vi "AlliGator All ROIs Phasor Analysis.vi"(8 "error in (no error)":errorcluster, 10 "New Plot Name":string, 11 "AlliGator Internal Variables DVR":refnum<data-value>) -> (0 "error out":errorcluster, 1 "Calibrated Phasor":T1, 2 "Phasor Plot":cluster{"g Array":dbl[], "s Array":dbl[]}, 3 "AlliGator Internal Variables DVR":refnum<data-value>, 4 "Calibrated Phase Lifetime":dbl[unit], 6 "Message":string)   [LabVIEW 2021, in "AlliGator Phasor Graph.lvlib"]
doc: "Non-interactive phasor analysis of all ROIs."
uses:
  AlliGator Phasor Graph.lvlib
  Internal Variables/AlliGator Internal Variables v2.ctl
  <vilib>/vision/Image Controls.llb/IMAQ Image.ctl
  Internal Variables/AlliGator Gate Image Set.ctl
  Files/AlliGator FLI Dataset Type.ctl
  Files/AlliGator Data Series Type.ctl
  Dual-Channel Datasets/AlliGator Dataset Channel.ctl
  Settings/AlliGator Gate Arithmetic.ctl
  Source Image/AlliGator Displayed Image.ctl
  Image/Named ROI Description.ctl
  AlliGator Decay Metadata v3.ctl
  Decay Analysis/Decay Preprocessing/AlliGator Decay Background Subtraction Info.ctl
  Decay Analysis/Decay Preprocessing/AlliGator Baseline Subtraction Method.ctl
  Graphs/XY Graph/XY Graph Plot Shift Parameters.ctl
  Graphs/XY Graph/XY Graph Plot Shift Method.ctl
  Decay Analysis/Decay Preprocessing/AlliGator Decay Extrapolation Parameters.ctl
  Phasor/Calibration Phasor (m, phi).ctl
  Phasor/Phasor Reference Series.ctl
  Phasor/Phasor Calibration Map v2.ctl
  Phasor/Phasor (g, s).ctl
  AlliGator Raw Phasor Plot Data v5.ctl
  Phasor/Phasor Standard Deviation Options.ctl
  Phasor Plot/AlliGator Phasor Multi-Harmonic Data.ctl
  Phasor/Phasor Harmonic Data.ctl
  Decay Fit Parameter Map/AlliGator Decay Fit Options & Parameters v4.ctl
  Fits/IRF(X)PSED/Decay Fit Options v4.ctl
  Fits/Decay Convolution/Decay Model.ctl
  Fits/Residual Type.ctl
  Fits/IRF(X)PSED/Fit Weights Type v2.ctl
  Fits/Non-linear Fitting Method v2.ctl
  Fits/Fit Calculation Method.ctl
  Fits/Non-linear Fitting Algorithm.ctl
  Decay Analysis/Decay Fit/AlliGator Decay Fit Parameter Constraints 2.ctl
  Fits/IRF(X)PSED/Decay Fit Parameters In List.ctl
  Fits/IRF(X)PSED/MLE Baseline Offset Type.ctl
  Decay Analysis/Decay Preprocessing/AlliGator Decay Preprocessing Parameters.ctl
  Fits/IRF(X)PSED/Decay Fit Parameters & Derived Quantities List v2.ctl
  Fits/IRF(X)PSED/Decay Fit Result Constraint.ctl
  Decay Fit Parameter Map/AlliGator Parameter Maps Data.ctl
  Globals, Variables, Constants/AlliGator Variables List.ctl
  Settings/AlliGator Settings List.ctl
  Rich Text Box/Text Format List.ctl
  Variant/Variant to Data/Variant to U16.vi
  <vilib>/Utility/error.llb/Error Cluster From Error Code.vi
  Globals, Variables, Constants/AlliGator Abort.vi
  <vilib>/ErrorRing/Error Ring.xnode
  Globals, Variables, Constants/AlliGator Globals, Variables & Constants.lvlib
  Image/Image.lvlib
  Decay Analysis/Decay Processing/AlliGator Decay Processing.lvlib
  Source Image/AlliGator Source Image.lvlib
  Phasor Calibration/AlliGator Phasor Calibration.lvlib
  Settings/AlliGator Settings.lvlib
  Phasor/Phasor.lvlib
  Strings/Strings.lvlib
  Time/Time.lvlib
  Decay Analysis/Decay Preprocessing/AlliGator Decay Preprocessing.lvlib
  Graphs/XY Graph/XY Graph Add-Ons.lvlib
  GUI/GUI.lvlib
  Notebook/Notebook.lvlib
  Error/Error.lvlib
  Variant/Variant to Data/Variant to Data.lvlib
  Utilities/Utilities.lvlib
  Files/AlliGator Files.lvlib
  Internal Variables/AlliGator Internal Variables.lvlib
  Phasor Plot/AlliGator Phasor Plot.lvlib
  Fits/Fits.lvlib
  Decay Analysis/Decay Fit/AlliGator Decay Fit.lvlib
  Dual-Channel Datasets/AlliGator Dual-Channel Datasets.lvlib
  Decay Fit Parameter Map/AlliGator Decay Fit Parameter Map.lvlib
panel:
  # "see the AlliGator License on the block diagram (Ctrl+E or Window:Show Block Diagram)"
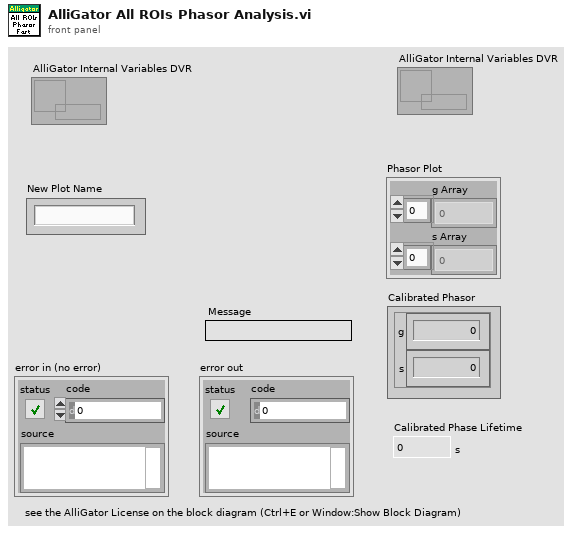
[diagram p1: front panel]
types:
  T1 = typedef "Phasor.lvlib/Phasor (g, s).ctl" = cluster{"g":dbl, "s":dbl}
  T2 = typedef "Phasor.lvlib/Phasor Standard Deviation Options.ctl" = cluster{"Compute Estimated SDV":bool, "# Replicas":u32, "Use Estimated Average Phasor":bool}
  T3 = typedef "AlliGator Settings.lvlib/AlliGator Settings List.ctl" = enum16{"GUI:Visible Settings Tab", "GUI:Last Run Version", "Source Image:Use Image Histogram for Contrast", "Source Image:Low Count Pixels Rejection Options", "Source Image:High Count Pixels Rejection Options", "Source Image:Use Image Brightness", "Source Image:Blend Overlay with Image Background", "Source Image:Use Fixed ROI Diameter", "Source Image:ROI Diameter", "Source Image:ROI Center Color", "Source Image:Peak Threshold", "Source Image:Intensity Threshold", "Source Image:Image Binning Options", "Source Image:Image Smoothing Options", "Source Image:Image Histogram Active", "Source Image:Invert Binary Mask", "Source Image:Hot Pixel Removal", "Source Image:Overlay Analyzed ROI Center", "Source Image:Auto-Adjust Contrast", "Source Image:Histogram Lower Percentile", "Source Image:Histogram Upper Percentile", "Source Image:Save Source Image", "Source Image:Scale Bar Options", "Source Image:Image Resolution (Pixel Size)", "Source Image:Flatfield Correction", "Source Image:Show Dead Left Columns Correction", "Source Image:Dead Left Columns Correction", "Source Image:Image Pre-Processing Operations Order", "Source Image:Overlay ROI Median", "Source Image:Median Overlay Color", "Data Information:Gate Width", "Data Information:Nanotime Gate Separation", "Data Information:Macrotime Gate Separation", "Data Information:Gate Step", "Data Information:# Gates", "Data Information:Gate Image Exposure", "Data Information:Gate Image Integration", "Data Information:Gates to Skip", "Data Information:Gates to Keep", "Data Information:Define Gates to", "Data Information:Channel Name", "Data Information:Available Channel Names", "Data Information:Channel Arithmetic", "Data Information:Background File Subtraction", "Data Information:Background File", "Data Information:Background Scaling Factor", "Data Information:Background Pile-up Correction", "Data Information:Background Pixel Well Capacity", "Data Information:Laser Period", "Data Information:SYNC Period", "Data Information:Pile-up Correction", "Data Information:Pixel Well Capacity", "Data Information:Dataset Scaling Factor", "Fluorescence Decay_Decay Pre-Processing:Reverse Gates", "Fluorescence Decay_Decay Pre-Processing:Verbose Decay Pre-Processing", "Fluorescence Decay_Decay Pre-Processing:Use Decay Pre-Processing", "Fluorescence Decay_Decay Pre-Processing:Background Subtraction", "Fluorescence Decay_Decay Pre-Processing:Background Definition Range", "Fluorescence Decay_Decay Pre-Processing:Baseline Subtraction Method", "Fluorescence Decay_Decay Pre-Processing:Decay Pre-Processing Operations Order", "Fluorescence Decay_Decay Pre-Processing:Smoothing Parameter", "Fluorescence Decay_Decay Pre-Processing:Shift Decay", "Fluorescence Decay_Decay Pre-Processing:Decay Shift Parameters", "Fluorescence Decay_Decay Pre-Processing:Fold Decay", "Fluorescence Decay_Decay Pre-Processing:# Folds", "Fluorescence Decay_Decay Pre-Processing:1-Normalize Decay", "Fluorescence Decay_Decay Pre-Processing:[0-1]-Normalize Decay", "Fluorescence Decay_Decay Pre-Processing:Smoothen Decay", "Fluorescence Decay_Decay Pre-Processing:Extrapolate Decay", "Fluorescence Decay_Decay Pre-Processing:Use Periodicity", "Fluorescence Decay_Decay Pre-Processing:Use Cursors", "Fluorescence Decay_Decay Pre-Processing:Tail Fraction", "Fluorescence Decay_Decay Pre-Processing:Head Fraction", "Fluorescence Decay_Decay Pre-Processing:Additional Points", "Fluorescence Decay_Decay Pre-Processing:Straighten Decay", "Fluorescence Decay_Decay Pre-Processing:Constant Background", "Fluorescence Decay_Decay Pre-Processing:Pixel-Normalize Decay", "Fluorescence Decay_Advanced Analysis:Extract IRF instead of Decay", "Fluorescence Decay_Advanced Analysis:IRF Extraction Options", "Fluorescence Decay_Advanced Analysis:IRF Optimization Options", "Fluorescence Decay_Advanced Analysis:Square Pulse Options", "Fluorescence Decay_Advanced Analysis:IRF Order", "Fluorescence Decay_Advanced Analysis:IRF Time Constants", "Fluorescence Decay_Advanced Analysis:Wavelet Analysis Options", "Fluorescence Decay_Advanced Analysis:Average Lifetime Options", "Fluorescence Decay_Fit Options:Fit Options", "Fluorescence Decay_Fit Options:Use Legacy Fitting Approach", "Fluorescence Decay_Fit Options:Use Data Information Laser Period", "Fluorescence Decay_Fit Parameters:Displayed Fit Parameters", "Fluorescence Decay_Fit Parameters:Fit Parameter Constraints", "Fluorescence Decay_Fit Parameters:Export Tabulated Results", "Fluorescence Decay_Fit Parameters:MLE Baseline Offset Type", "Fluorescence Decay_Fit Parameters:MLE Baseline Offset", "Fluorescence Decay_Fit Parameters:Guess Parameter Names", "Fluorescence Decay_Fit Parameters:Guess Parameter Values", "Fluorescence Decay_Fit Parameters:Guess Parameters Options", "Fluorescence Decay_Fit Parameters:Optimal Offset Selection Criterion", "Fluorescence Decay_Styles:Show Last Decay Only", "Fluorescence Decay_Styles:Decay Graph Color Array", "Fluorescence Decay:Decay Graph Active", "Fluorescence Decay Statistics:Min Peak Value", "Fluorescence Decay Statistics:Reject Low Decay Peak Pixels", "Fluorescence Decay Statistics:Reject High Decay Peak Pixels", "Fluorescence Decay Statistics:Max Peak Value", "Time Traces:Use File Timestamp", "Time Traces:Time Step", "Time Traces:Use Intensity Correction File", "Time Traces:Intensity Correction File", "Phasor Plot:Phasor Plot Smoothing Options", "Phasor Plot:Phasor Plot Size", "Phasor Plot:Phasor Plot Graphics Options", "Phasor Plot:Cumulative Phasor Plot", "Phasor Plot:Use Phasor Brightness", "Phasor Plot:Blend Overlay with Phasor Background", "Phasor Plot:Save Phasor Plot", "Phasor Plot:Show References", "Phasor Plot:Phasor Ratio Decay Range", "Phasor Plot:Exponential Fading", "Phasor Plot:Phasor Ratio Reference Colors", "Phasor Plot:Reference Radius", "Phasor Plot:Show Color Map Vertices", "Phasor Plot:Phasor Plot Active", "Phasor Plot:Phasor Ratio Color Map Type", "Phasor Plot:Phasor Ratio Color Map", "Phasor Plot:Phasor Ratio Display Range", "Phasor Plot:Selected Image ROI(s)", "Phasor Plot:All Image ROIs", "Phasor Plot:Selected Phasor Plot ROI(s)", "Phasor Plot:All Phasor Plot ROIs", "Phasor Plot:Phasor Ratio Color-Coded Quantity", "Phasor Plot:Store Phasor Harmonics", "Phasor Plot:Draw Reference Segment", "Phasor Plot:User-Defined Quantity", "Phasor Plot:Color Scale High Color", "Phasor Plot:Color Scale Low Color", "Phasor Plot:Intensity-weighted Phasor Plot", "Phasor Graph:Phasor Frequency", "Phasor Graph:Phasor Ratio Type", "Phasor Graph:Pixel-level Phasor Computation", "Phasor Graph:Save Phasor Graph", "Phasor Graph:Phasor Graph Active", "Phasor Graph:Phasor SDV Options", "Phasor Graph:Intensity-weighted Phasor Graph", "Phasor Graph:Define Shortest Lifetime as", "Phasor Calibration:Use Backup Calibration if needed", "Phasor Calibration:Backup Calibration Type", "Phasor Calibration:Calibration Type", "Phasor Calibration:Calibration Lifetime", "Phasor Calibration:Calibration Map Algorithm", "Single-Exponential Phasor Locus (SEPL):Gate Parameters", "Single-Exponential Phasor Locus (SEPL):User-defined Gate", "Single-Exponential Phasor Locus (SEPL):User-defined IRF", "Single-Exponential Phasor Locus (SEPL):Phasor Parameters", "Single-Exponential Phasor Locus (SEPL):Decay & IRF Parameters", "Single-Exponential Phasor Locus (SEPL):Display Parameters", "Lifetime Analysis:Decay Analysis Parameters", "Lifetime Analysis:Lifetime Map Active", "Plugins:Python Settings", "Miscellaneous:Verbose Mode", "Miscellaneous:Beep after Script", "Miscellaneous:Saved Image File Format", "Miscellaneous:Exported Gate Image Settings", "Miscellaneous:Include Loading in Timing", "Miscellaneous:Verbose Settings Mode", "Miscellaneous:Histogram Options", "Miscellaneous:Beep on Error", "Miscellaneous:# Logical Processors Used", "Miscellaneous:ROI Description Max Characters", "Miscellaneous:Verbose Error Mode", "Miscellaneous:Transparent Mask Color"}
  T4 = typedef "AlliGator Globals, Variables & Constants.lvlib/AlliGator Variables List.ctl" = enum16{"---- GUI ----", "GUI:Initialization Status", "GUI:State Indicators Refnum", "GUI:Original AlliGator Menu Items", "GUI:Current Action Loop State", "GUI:Script in progress", "GUI:Playback", "GUI:Loop Playback", "GUI:Search ROI Used", "GUI:Search ROI", "Decay Graph Max Legend Size", "Intensity Graph Max Legend Size", "Decay Statistics Graph Max Legend Size", "Phasor Graph Max Legend Size", "Phasor Ratio Graph Max Legend Size", "Lifetime Graph Max Legend Size", "---- Files ----", "Files:Export Dataset Frames as Individual Files", "Files:Show Batch Export Help Balloons", "Files:Frames in Dataset", "Files:ptu File Frame Start Indices", "Files:Current Frame in Dataset", "Files:Current Frame Timestamp", "Files:Dataset Loaded", "Files:Dataset Metadata", "Files:Dataset Channel", "Files:Dataset Data Description", "Files:Background Dataset Metadata", "Files:Background Dataset Channel", "Files:Background Dataset Data Description", "Files:Background File Subtraction", "Files:Background File Path", "Files:Background File Pile-up Correction", "Files:Background File Pixel Well Capacity", "Files:Background File Scaling Factor", "Files:Current Dataset Load Settings", "Files:Dataset Path", "Files:ICCD-specific Information", "Files:Macrotime Gate Separation", "------ Python Plugins ------", "Python Plugins:Information", "Python Plugins:Python Session", "Python Plugins:Valid Python Session?", "---- Source Image ----", "Source Image:ROIs", "Source Image:Current ROI", "Source Image:ROI Event Refnum", "X_Source Image:Display Range", "X_Source Image:Palette Information", "X_Source Image:Type of Displayed Image", "X_Time Gate Slider", "Source Image:Palette List", "Source Image:Scale", "Source Image:ROI Overlay Color", "Source Image:Overlay to Erase", "Source Image:Is Displayed Image Accumulated", "Source Image:White Light Image Modified", "Source Image:Mask Image Modified", "---- Image Profile Window ----", "Image Profile:Window Event Refnum", "Image Profile:IntensityType", "Image Profile:Intensity Average Type", "Image Profile:Intensity-weighted SDV", "Image Profile:Box Profile Type", "Image Profile:Window Open", "Image Profile:Plotted Fit Parameter", "------ Phasor Graph -------", "Phasor Graph:Show Line", "---- Phasor Plot ---", "Phasor Plot:Parameters Changed", "Phasor Plot:FLI Dataset Modified since last Calculation", "Phasor Harmonics Data", "Selected Phasor Harmonics", "Phasor Harmonic Manager Event Refnum", "Phasor Plot:ROIs", "Phasor Plot:Current ROI", "Phasor Plot:ROI Event Refnum", "Phasor Plot:Image Reference Points", "Phasor Plot:Computed", "Phasor Plot:Palette Information", "Phasor Plot:Palette List", "Phasor Plot:Phasor Ratio Palette Information", "Phasor Plot:Phasor Ratio Palette List", "Phasor Plot:Image Scale", "Phasor Plot:Image Overlay to Erase", "Phasor Plot:Image Elements to Update", "Phasor Plot:Current Calculation Parameters", "Phasor Plot:Current Calibration Options", "Phasor Plot:Reset Cumulated Phasor Plot", "Phasor Plot:Reference 1", "Phasor Plot:Lifetime Reference 1", "Phasor Plot:Reference 1 Frequency", "Phasor Plot:Reference 2", "Phasor Plot:Lifetime Reference 2", "Phasor Plot:Reference 2 Frequency", "---- Decay Analysis ----", "Number of Selected Decays to Fit", "LS Fit Results", "LAR Fit Results", "BS Fit Results", "Last Decay Max - Min", "Best Fit Parameters", "Best Fit Parameter Names", "Actual Size X", "Actual Size Y", "Binning X", "Binning Y", "Actual # Gates", "Dataset Number", "Gates to...", "Gates Skipped", "Gates to keep", "Gate Step", "Gate Separation", "Reversed Gates", "Pile-up Correction", "Pixel Well Capacity", "Background Subtracted", "Background Subtraction Method", "Background Definition Range", "Background File (deprecated)", "Number of Dataset Accumulated", "Array of Accumulated Dataset Paths", "Do Averaged Datasets", "Destination File Path", "Process Plot Target", "Use 1/D as Phasor Frequency", "---- Decay Fit Parameter Map -----", "Decay Fit Parameter Map:Palette Information", "Decay Fit Parameter Map:Palette List", "Decay Fit Parameter Map:X Resolution", "Decay Fit Parameter Map:Y Resolution", "Decay Fit Parameter Map:Use Decay Fit Result Constraints", "Decay Fit Parameter Map:Decay Fit Result Constraints", "Decay Fit Parameter Map:Decay Fit Result Constraints Applied", "---- Parameter Map ----", "Parameter Map:Palette Information", "Parameter Map:Palette List", "------- Local Decay Window ---------", "Local Decay Graph Window:Event Refnum", "Local Decay Graph Window:Use normalized IRF for convolution", "----- Miscellaneous ----", "Misc:Skippable Dialog Windows Status"}
  T5 = typedef "IMAQ Image.ctl" = refnum<image>
  T6 = typedef "Image.lvlib/Named ROI Description.ctl" = cluster{"ROI Descriptor":T7, "ROI Name":string, "Overlay Color":u32}
  T7 = typedef "ROI Descriptor" = cluster{"Global Rectangle":i32[], "Contours":cluster{"ID":enum32{"External", "Internal"}, "Type":u32, "Coordinates":i32[]}[]}
  T8 = typedef "Notebook.lvlib/Text Format List.ctl" = enum16{"Message", "Result", "Error", "Setting", "Verbose", "Warning"}
  T9 = typedef "AlliGator Phasor Graph.lvlib/AlliGator Raw Phasor Plot Data v5.ctl" = cluster{"Phasor Plot Name":string, "Raw Phasor Plot":T1[], "Phasor Frequency":dbl[unit], "[Decay Metadata]":T10[], "Raw Phasor Plot SDV":T1[], "Phasor SDV Options":T2, "[Calibration Phasor]":T16[], "Intensity Array":dbl[]}
  T10 = typedef "AlliGator Phasor Graph.lvlib/AlliGator Decay Metadata v3.ctl" = cluster{"ROI Descriptor":T7, "ROI Center":cluster{"X":i32, "Y":i32}, "Decay Background Subtraction Info":T11, "Decay Reverted":bool, "Decay Smoothened":bool, "Decay Straightened":bool, "Fitted Tau (Decay Straightening)":dbl, "Decay Shift Parameters":T13, "Decay Shifted":bool, "Decay Extrapolated":bool, "Decay Extrapolation Parameters":T15, "Decay Normalized":bool, "Fold Decay":bool, "# Folds":u32}
  T11 = typedef "AlliGator Decay Preprocessing.lvlib/AlliGator Decay Background Subtraction Info.ctl" = cluster{"Laser Period":dbl[unit], "Gate Duration":dbl[unit], "Baseline Subtraction Method":T12, "Background Definition Range":cluster{"Min Gate":dbl[unit], "Max Gate":dbl[unit]}, "Total Intensity w/o Bkgd Subtraction":dbl, "Bkgd-subtracted Intensity (exp)":dbl, "# Data Points":i32, "Background/Gate":dbl, "Fitted Lifetime":dbl[unit], "Bkgd-subtracted Intensity (theo)":dbl}
  T12 = typedef "AlliGator Decay Preprocessing.lvlib/AlliGator Baseline Subtraction Method.ctl" = enum16{"Mean", "Min", "Square Gated Single-Exponential", "File", "Constant"}
  T13 = typedef "XY Graph Add-Ons.lvlib/XY Graph Plot Shift Parameters.ctl" = cluster{"Type":T14, "Shift":dbl[unit], "Threshold":dbl, "Rotate":bool}
  T14 = typedef "XY Graph Add-Ons.lvlib/XY Graph Plot Shift Method.ctl" = enum16{"Default", "CFD", "Threshold", "Cross-Correlation"}
  T15 = typedef "AlliGator Decay Preprocessing.lvlib/AlliGator Decay Extrapolation Parameters.ctl" = cluster{"Additional Points":u32, "Head Fraction":dbl, "Fitted Tau":dbl, "Use Periodicity":bool, "Use Cursors":bool, "Tail Fraction":dbl}
  T16 = typedef "Phasor.lvlib/Calibration Phasor (m, phi).ctl" = cluster{"m":dbl, "phi":dbl, "Phasor Frequency":dbl[unit], "Reference Lifetime":dbl[unit]}
  T17 = typedef "AlliGator Internal Variables.lvlib/AlliGator Internal Variables v2.ctl" = cluster{"----------------------------- Images -----------------------------":u8, "Displayed Image":T5, "White Light Image":T5, "Mask Image":T5, "ROI Mask Image":T5, "Current Dataset Images 1":T18, "Background Dataset Images 1":T18, "Current Dataset Images 2":T18, "Background Dataset Images 2":T18, "Current Dataset Arithmetic Images":T18, "Accumulated Dataset Images 1":T18, "Accumulated Dataset Images 2":T18, "Accumulated Dataset Arithmetic Images":T18, "----------------------------- File Paths -----------------------------":u8, "Phasor Plot Image":T5, "Decay Fit Parameter Map Image":T5, "Parameter Map Image":T5, "Single Data Point Path":path, "White Light Image Path":path, "Mask Image Path":path, "Time-Series Folder":path, "[Time-Series Paths]":path[], "----------------------------- FLI Dataset -----------------------------":u8, "Current Dataset":i32, "Single Dataset Type":T19, "Current Folder":string, "AlliGator Data Series Type":T20, "# Datasets":i32, "Dual-Channel Dataset":bool, "Selected Channel Name":string, "Dataset Channel":T21, "Channel Arithmetic":T22, "Dual-Channel Background Dataset":bool, "Background Channel":T21, "Dual-Channel Accumulated Dataset":bool, "Start Time":dbl, "[Time-Series Timestamps]":dbl[], "[Intensity Corrections]":dbl[], "Time Series Script":bool, "Type of Displayed Image":T23, "Gate Image Slide":u16, "# Gates":i32, "ROIs":T6[], "----------------------------- Decays -----------------------------":u8, "ROI Decay":cluster{"t Array":dbl[], "I Array":dbl[]}, "Valid Decay":bool, "Decay  Metadata":T10, "Reference Decay Plot Name":string, "Reference Decay":cluster{"t Array":dbl[], "I Array":dbl[]}, "Decay Shift Plot":cluster{"Time Stamps":dbl[], "Decay Shifts":dbl[]}, "[Decays Max Values]":sgl[], "[Decays Min Values]":sgl[], "----------------------------- Calibration -----------------------------":u8, "Calibration Phasor":T16, "Calibration Phasor Series":T24, "Phasor Calibration Map":T25, "Calibration Map MD5 Digest":string, "----------------------------- Phasor Graph -----------------------------":u8, "Last Raw Phasor":T1, "Last Calibrated Phasor":T1, "Last Calibrated Phasor SDV":T1, "Phasor Graph:Phasor Plot":cluster{"g Array":dbl[], "s Array":dbl[]}, "Phasor Graph:Phasor SDV Plot":cluster{"g Array":dbl[], "s Array":dbl[]}, "[Phasor Graph:Raw Phasor Plots]":T9[], "Phasor Plot locked to Ref 1":i32, "[Phasor Plot(s) locked to Ref 1]":i32[], "[Phasor Plot(s) locked to Ref 2]":i32[], "[Pixel Phasors]":T1[], "----------------------------- Phasor Plot -----------------------------":u8, "[[Sum Image]]":dbl[][], "[[CSG Phasors]]":csg[][], "[[Valid Pixel?]]":bool[][], "[[Phasor Ratios]]":dbl[][], "[[Average Lifetimes]]":dbl[][], "Amplitude Weighted Average Lifetime":bool, "I/m/phi Dataset":cluster{"I/m/phi Dataset?":bool, "Base Frequency":dbl[unit], "Harmonic Orders":u8[]}, "Multi Phasor Plot Data":T26, "----------------------------- Decay Fit Parameter Map -----------------------------":u8, "Decay Fit Options & Parameters":T28, "Fit Options: Decay Preprocessing Parameters":T39, "Fit Options: Reference Decay":cluster{"t Array":dbl[], "I Array":dbl[]}, "Is Full Image Parameters Map":bool, "Is Single-Pixels Parameters Map":bool, "NLSF Parameters Map X Resolution":i32, "NLSF Parameters Map Y Resolution":i32, "[Single Decay Fit Parameters]":dbl[], "Fit Model":T30, "[[Multiple Decays Fit Parameters]]":dbl[][], "[[Multiple Decays Fit Parameter SDVs]]":dbl[][], "[[IRFs]]":dbl[][], "[ROI Descriptors]":T7[], "IRF Array Time Axis":dbl[], "Decay Array Time Axis":dbl[], "[Decay Fit Parameter Names]":T40[], "[Decay Sum]":dbl[], "Array of Decay Fit Result Constraints":T41[], "Selected ROIs Array":bool[], "----------------------------- Parameter Maps -----------------------------":u8, "[Map Set Names]":string[], "[Parameter Maps]":T42[], "[[User-defined Quantities]]":dbl[][], "User-defined Quantity":string}
  T18 = typedef "AlliGator Internal Variables.lvlib/AlliGator Gate Image Set.ctl" = cluster{"SGL Gate Images":T5[], "SGL Sum Image":T5, "SGL Max Image":T5, "SGL Min Image":T5}
  T19 = typedef "AlliGator Files.lvlib/AlliGator FLI Dataset Type.ctl" = enum16{"HDF5 FLI Dataset", "Gate Image Folder", ".sdt FLI Dataset (Becker & Hickl)", ".ptu FLI Dataset (PicoQuant)", "SS1 FLI Dataset", "SS2 FLI Dataset", "I/m/phi Dataset", ".bin FLI Dataset (PicoQuant Binned)", ".bin FLI Dataset (Piccolo Binned)", ".mat FLI Dataset"}
  T20 = typedef "AlliGator Files.lvlib/AlliGator Data Series Type.ctl" = enum16{"Not a Supported Series", "Gate Images Folder Series", "SwissSPAD 2 Dataset Series", "B&H FLI Dataset Series", "PicoQuant PTU FLI Dataset Series", "PicoQuant BIN FLI Dataset Series", "Piccolo hist BIN FLI Dataset Series", "HDF5 FLI Dataset Series"}
  T21 = typedef "AlliGator Dual-Channel Datasets.lvlib/AlliGator Dataset Channel.ctl" = enum16{"G2", "INT"}
  T22 = typedef "AlliGator Settings.lvlib/AlliGator Gate Arithmetic.ctl" = enum16{"None", "INT-G2", "G2/INT*<INT>", "(1 - G2/INT)*<INT>"}
  T23 = typedef "AlliGator Source Image.lvlib/AlliGator Displayed Image.ctl" = enum16{"Single Gate", "Sum of All Gates", "Max of All Gates", "Min of All Gates", "-", "White Ligth Image", "Mask Image"}
  T24 = typedef "Phasor.lvlib/Phasor Reference Series.ctl" = cluster{"m Array":dbl[], "phi Array":dbl[], "Phasor Frequency":dbl[unit], "Calibration Lifetime":dbl[unit]}
  T25 = typedef "Phasor.lvlib/Phasor Calibration Map v2.ctl" = cluster{"Phasor Frequency":dbl[unit], "Calibration Lifetime":dbl[unit], "ROI Centers":cluster{"X":i32, "Y":i32}[], "ROI Descriptors":T7[], "Map Resolution X":i32, "Map Resolution Y":i32, "z Array":cdb[]}
  T26 = typedef "AlliGator Phasor Plot.lvlib/AlliGator Phasor Multi-Harmonic Data.ctl" = cluster{"Base Frequency":dbl[unit], "# Harmonics":u8, "Harmonic Orders":u8[], "Phasor Plot Settings Checksum":u64, "Phasor Harmonic Data Array":T27[]}
  T27 = typedef "Phasor.lvlib/Phasor Harmonic Data.ctl" = cluster{"Phasor Harmonic Name":string, "Phasor Plot Settings Checksum":u64, "Phasor Frequency":dbl[unit], "Base Frequency":dbl[unit], "Harmonic Order":u8, "Phasor Plot Parameters":string, "Phasor Array [[CSG]]":csg[][], "Dataset File Path":path}
  T28 = typedef "AlliGator Decay Fit Parameter Map.lvlib/AlliGator Decay Fit Options & Parameters v4.ctl" = cluster{"SYNC Period":dbl[unit], "Fit Options":T29, "Fit Parameter Constraints":T36[], "MLE Baseline Offset":dbl, "MLE Baseline Offset Type":T38}
  T29 = typedef "Fits.lvlib/Decay Fit Options v4.ctl" = cluster{"Show Fit Residuals":bool, "Fit Model":T30, "Residual Type":T31, "Max Decay Percentile":dbl, "Min Decay Percentile":dbl, "Show Full Decay":bool, "Weights":T32, "Fitting Method":T33, "Compute Parameter Uncertainties":bool, "Periodic Boundaries":bool, "Model Calculation":T34, "Period":dbl[unit], "Termination Criteria":cluster{"Max Iterations":i32, "Max Function Calls":i32, "Max Time":dbl[unit], "Function Tolerance":dbl, "Parameter Tolerance":dbl, "Gradient Tolerance":dbl, "Min Lambda":dbl, "Max Lambda":dbl, "Initial Tick Count":u32}, "Offset Resolution":dbl[unit], "Use Local IRF":bool, "Fitting Algorithm":T35, "Show Confidence Interval ":bool, "Confidence Level":dbl}
  T30 = typedef "Fits.lvlib/Decay Model.ctl" = enum16{"1-Exponential", "2-Exponentials"}
  T31 = typedef "Fits.lvlib/Residual Type.ctl" = enum16{"Standard", "Normalized", "Reduced"}
  T32 = typedef "Fits.lvlib/Fit Weights Type v2.ctl" = enum16{"Unweighted", "1/Variance (Neyman)", "1/Variance (Pearson)", "Best of All"}
  T33 = typedef "Fits.lvlib/Non-linear Fitting Method v2.ctl" = enum16{"Least Square", "Least Absolute Residual", "Bisquare", "MLE", "-", "Best of All"}
  T34 = typedef "Fits.lvlib/Fit Calculation Method.ctl" = enum16{"Simulation", "Convolution", "Integration"}
  T35 = typedef "Fits.lvlib/Non-linear Fitting Algorithm.ctl" = enum16{"Levenberg-Marquardt", "Trust-Region Dogleg"}
  T36 = typedef "AlliGator Decay Fit.lvlib/AlliGator Decay Fit Parameter Constraints 2.ctl" = cluster{"Fit Parameter":T37, "Min Value":dbl, "Max Value":dbl, "Global":bool, "Used":bool}
  T37 = typedef "Fits.lvlib/Decay Fit Parameters In List.ctl" = enum16{"Offset", "Baseline", "A_1", "tau_1", "A_2", "tau_2"}
  T38 = typedef "Fits.lvlib/MLE Baseline Offset Type.ctl" = enum32{"Absolute", "Percentage"}
  T39 = typedef "AlliGator Decay Preprocessing.lvlib/AlliGator Decay Preprocessing Parameters.ctl" = cluster{"Background Subtraction":bool, "Straighten Decay":bool, "Reverse Gates":bool, "1-Normalized Decay":bool, "Smoothen Decay":bool, "Smoothing Parameter":dbl, "Shift Decay":bool, "Decay Shift Parameters":T13, "Extrapolate Decay":bool, "Additional Points":u32, "Head Fraction":dbl, "Pixel-Normalize Decay":bool, "Use Periodicity":bool, "Use Cursors":bool, "Tail Fraction":dbl, "Use Decay Pre-Processing":bool, "Fold Decay":bool, "# Folds":u32, "[0-1]-Normalized Decay":bool}
  T40 = typedef "Fits.lvlib/Decay Fit Parameters & Derived Quantities List v2.ctl" = enum16{"Offset", "Baseline", "A_1", "tau_1", "A_2", "tau_2", "<tau>_a", "f1_a", "f2_a", "<tau>_i", "f1_i", "f2_i", "-", "R^2", "Chi^2"}
  T41 = typedef "Fits.lvlib/Decay Fit Result Constraint.ctl" = cluster{"Fit Parameter":enum16{"Offset", "Baseline", "A_1", "tau_1", "A_2", "tau_2", "<tau>_a", "f1_a", "f2_a", "<tau>_i", "f1_i", "f2_i", "-", "R^2", "Chi^2", "Max Relative Residual", "<Residual ACF>", "Residual ACF SDV", "tau_2/tau_1"}, "Min Value":dbl, "Max Value":dbl, "Use Constraint":bool}
  T42 = typedef "AlliGator Decay Fit Parameter Map.lvlib/AlliGator Parameter Maps Data.ctl" = cluster{"Map Set Name":string, "[Parameter Names]":string[], "[[Parameters]]":dbl[][], "[[Parameter SDVs]]":dbl[][], "Decay Array Time Axis":dbl[], "[[IRFs]]":dbl[][], "IRF Array Time Axis":dbl[], "X Resolution":i32, "Y Resolution":i32, "Intensity Array":dbl[]}
  T43 = cluster{"Decay Peak Constraint":bool, "Min":dbl, "Max":dbl}
  T44 = typedef "Phasor.lvlib/Phasor Calibration Type.ctl" = enum16{"None", "Single Phasor", "Phasor Series", "Phasor Map"}
  T45 = cluster{"Use Backup Calibration if needed?":bool, "Calibration Type":T44}
  T46 = typedef "AlliGator Settings.lvlib/AlliGator Pixel Counts Constraints.ctl" = cluster{"High Count Pixels Rejection Options":T47, "Low Count Pixels Rejection Options":T48}
  T47 = typedef "AlliGator Settings.lvlib/AlliGator High Count Pixels Rejection Options.ctl" = cluster{"Background High Threshold Factor":dbl, "Fixed High Background Threshold":dbl, "Reject High Count Pixels":bool, "High Percentile":dbl}
  T48 = typedef "AlliGator Settings.lvlib/AlliGator Low Count Pixels Rejection Options.ctl" = cluster{"Background Low Threshold Factor":dbl, "Fixed Low Background Threshold":dbl, "Reject Low Count Pixels":bool, "Low Percentile":dbl}
  T49 = cluster{"t Axis":dbl[], "ROI Intensity Array":dbl[]}
  T50 = typedef "Rich Text Box.lvlib/Text Formatting.ctl" = cluster{"Font":string, "Text Color":T51, "Background Color":T51, "Style":T52, "Font Size":dbl, "Alignment":T53}
  T51 = typedef "Rich Text Box.lvlib/Text Colors.ctl" = enum16{"Unchanged", "Black", "Blue", "Cyan", "Maroon", "Gray", "Violet", "Green", "Light Green", "Orange", "Yellow", "Magenta", "Red", "White"}
  T52 = typedef "Rich Text Box.lvlib/Text Style.ctl" = enum16{"Regular", "Bold", "Italic", "Underline", "Strikeout"}
  T53 = typedef "Rich Text Box.lvlib/Text Alignment.ctl" = enum16{"Left", "Right", "Center"}
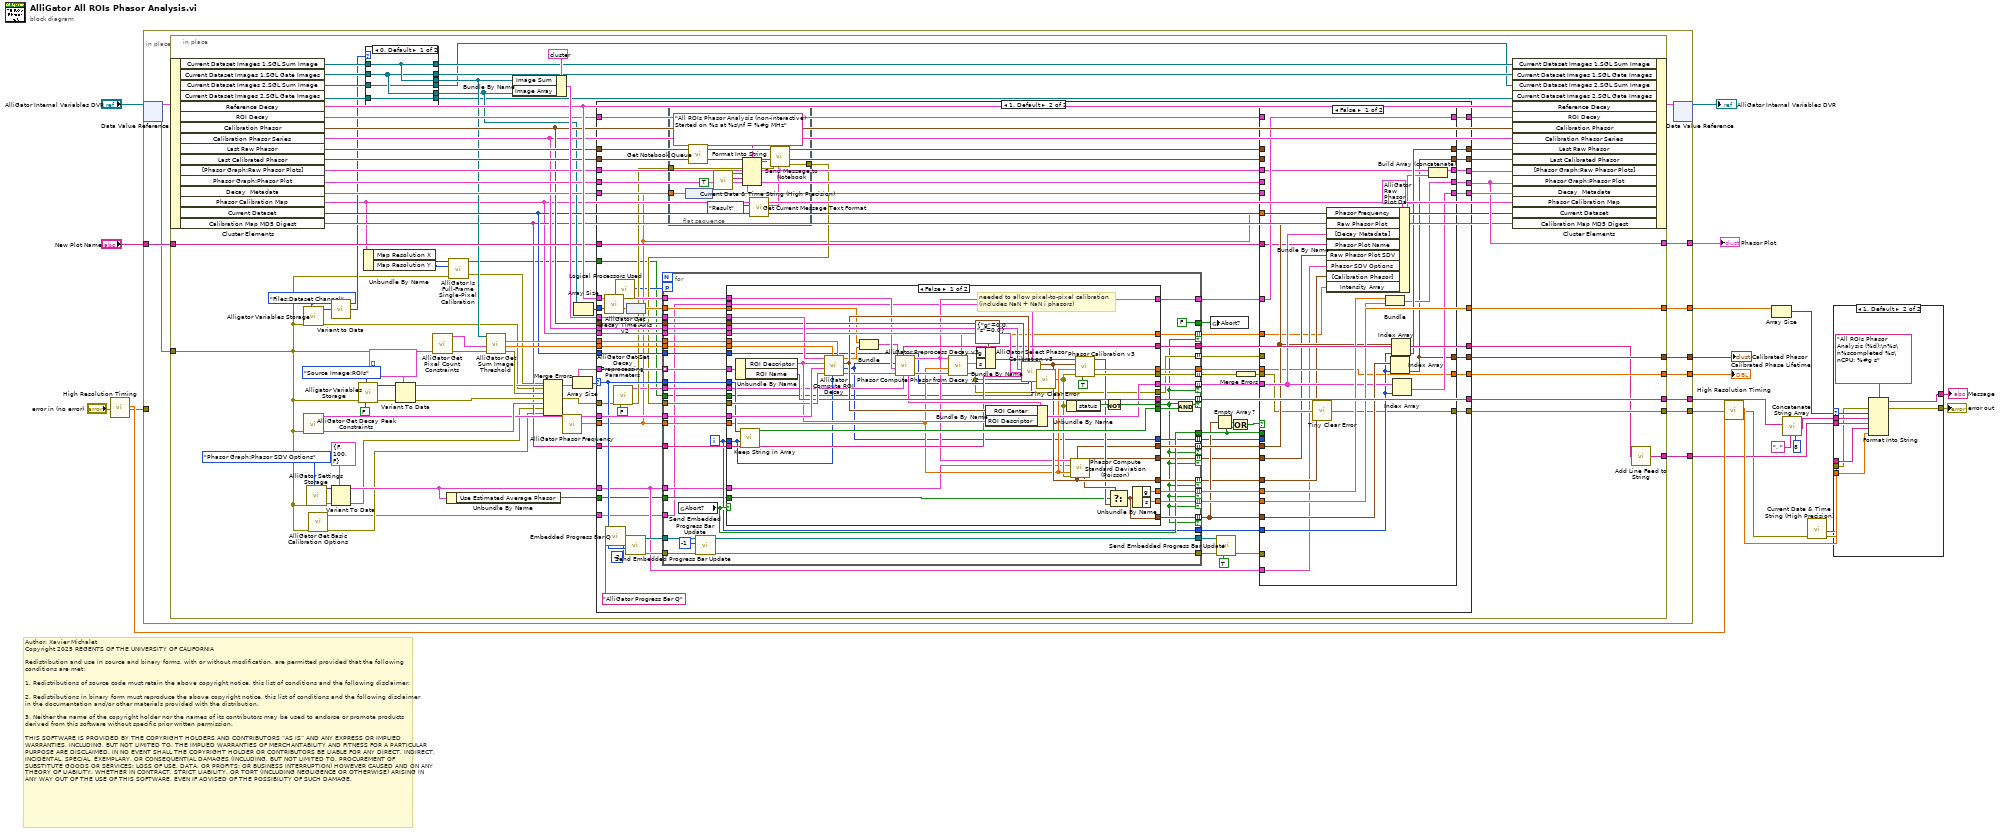
[diagram p0: block diagram]
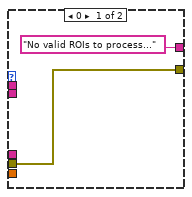
[diagram p2: hidden frame]
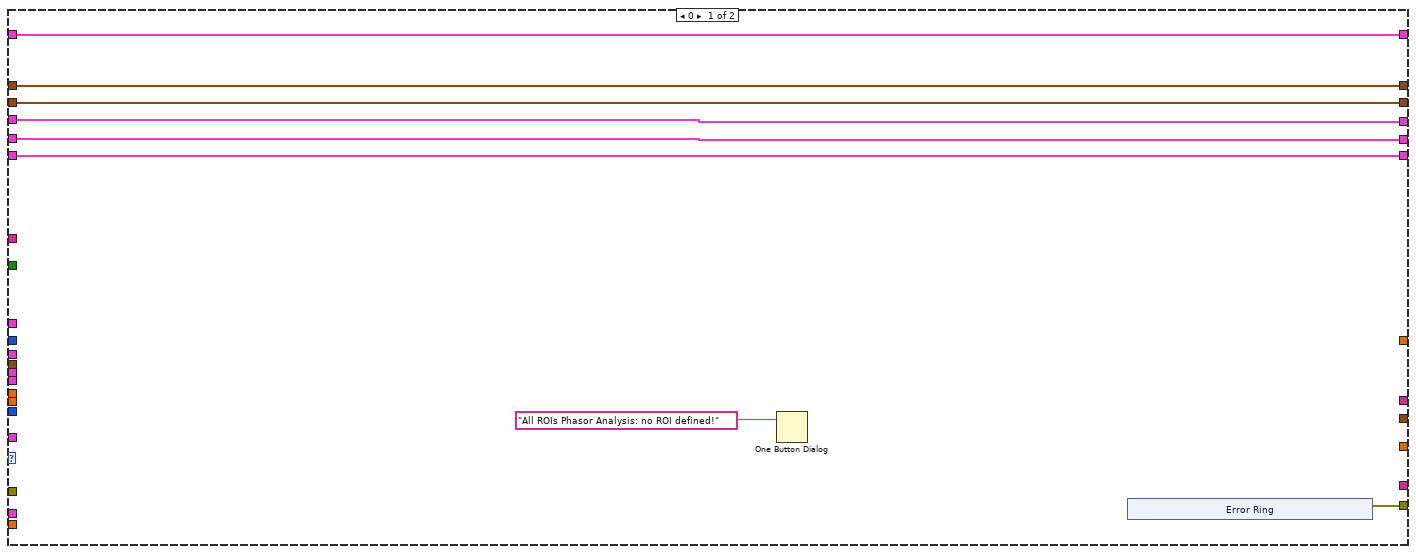
[diagram p4: hidden frame]
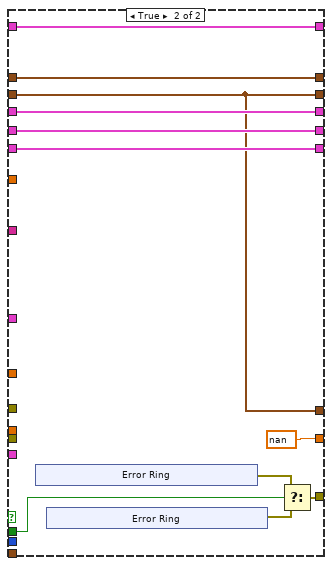
[diagram p5: hidden frame]
diagram:
  # "Author: Xavier Michalet\nCopyright 2025 REGENTS OF THE UNIVERSITY OF CALIFORNIA\n\nRedistribution and use in source and binary forms, with or without modification, are permitted provided that the following conditions are met:\n\n1. Redistributions of source code must retain the above copyright notice, this list of conditions and the following disclaimer.\n\n2. Redistributions in binary form must reproduce the above copyright notice, this list of conditions and the following disclaimer in the documentation and/or other materials provided with the distribution.\n\n3. Neither the name of the copyright holder nor the names of its contributors may be used to endorse or promote products derived from this software without specific prior written permission.\n\nTHIS SOFTWARE IS PROVIDED BY THE COPYRIGHT HOLDERS AND CONTRIBUTORS “AS IS” AND ANY EXPRESS OR IMPLIED WARRANTIES, INCLUDING, BUT NOT LIMITED TO, THE IMPLIED WARRANTIES OF MERCHANTABILITY AND FITNESS FOR A PARTICULAR PURPOSE ARE DISCLAIMED. IN NO EVENT SHALL THE COPYRIGHT HOLDER OR CONTRIBUTORS BE LIABLE FOR ANY DIRECT, INDIRECT, INCIDENTAL, SPECIAL, EXEMPLARY, OR CONSEQUENTIAL DAMAGES (INCLUDING, BUT NOT LIMITED TO, PROCUREMENT OF SUBSTITUTE GOODS OR SERVICES; LOSS OF USE, DATA, OR PROFITS; OR BUSINESS INTERRUPTION) HOWEVER CAUSED AND ON ANY THEORY OF LIABILITY, WHETHER IN CONTRACT, STRICT LIABILITY, OR TORT (INCLUDING NEGLIGENCE OR OTHERWISE) ARISING IN ANY WAY OUT OF THE USE OF THIS SOFTWARE, EVEN IF ADVISED OF THE POSSIBILITY OF SUCH DAMAGE."
  n1 = call "High Resolution Timing.vi"("Error In"="error in (no error)") -> ("elapsed (relative) seconds"=w13:dbl, "Error Out"=w7:errorcluster)  [unwired: 16 in, 1 out]
  n2 = in-place {
    in-place-border: [w32] -> w4
    in-place-border: [w31] -> w20
    in-place-border: "New Plot Name" -> [w30]
    in-place-border: [w29] -> w18
    in-place-border: [w28] -> w17
    in-place-border: [w27] -> w9
    in-place-border: w7 -> [_]
    in-place-border: [w25] -> w6
    in-place-border: [w24] -> w3
    n3 = in-place-dvr #1("AlliGator Internal Variables DVR") -> (w34:T17, w26:errorcluster)
    n4 = in-place {
      in-place-border: w26 -> [w37]
      in-place-border: [w92] -> w32
      in-place-border: [w80] -> w31
      in-place-border: w30 -> [w79]
      in-place-border: [w78] -> w29
      in-place-border: [w77] -> w28
      in-place-border: [w76] -> w27
      in-place-border: [w74] -> w25
      in-place-border: [w67] -> w24
      n5 = in-place-cluster #2(w34) -> ("Current Dataset Images 1.SGL Sum Image"=w61:T5, "Current Dataset Images 1.SGL Gate Images"=w60:T5[], "Current Dataset Images 2.SGL Sum Image"=w64:T5, "Current Dataset Images 2.SGL Gate Images"=w63:T5[], "Reference Decay"=w93:cluster{"t Array":dbl[], "I Array":dbl[]}, "ROI Decay"=w82:cluster{"t Array":dbl[], "I Array":dbl[]}, "Calibration Phasor"=w73:T16, "Calibration Phasor Series"=w72:T24, "Last Raw Phasor"=w91:T1, "Last Calibrated Phasor"=w89:T1, "[Phasor Graph:Raw Phasor Plots]"=w87:T9[], "Phasor Graph:Phasor Plot"=w85:cluster{"g Array":dbl[], "s Array":dbl[]}, "Decay  Metadata"=w84:T10, "Phasor Calibration Map"=w40:T25, "Current Dataset"=w70:i32, "Calibration Map MD5 Digest"=w59:string)
      n6 = call "Alligator Variables Storage.vi"("AlliGator Variable"=AlliGator_Variables_List."Files:Dataset Channel" ("Alligator Variable"), "Error In"=w37) -> ("Error Out"=w41:errorcluster, "Data out"=w57:variant)  [unwired: 7 in, 1 out]
      n7 = call "AlliGator Get Decay Peak Constraints.vi"("error in (no error)"=w37) -> ("Error Out"=w97:errorcluster, "Decay Peak Constraints"=w96:T43)  [unwired: 9 in]
      n8 = call "AlliGator Settings Storage.vi"("AlliGator Settings List"=AlliGator_Settings_List."Phasor Graph:Phasor SDV Options", "Error In"=w37) -> ("Error Out"=w55:errorcluster, "Variant Data out"=w54:variant)  [unwired: 8 in]
      n9 = call "AlliGator Get Basic Calibration Options.vi"("error in (no error)"=w37) -> ("error out"=w43:errorcluster, "Basic Calibration Options"=w42:T45)  [unwired: 9 in]
      n10 = call-poly "Variant to Data.vi"("Variant"=w57) -> ("U16 Value"=w56:u16)  [unwired: 8 in]
      n11 = Variant To Data(error in=w55, type=T2 {"Compute Estimated SDV"=FALSE, "# Replicas"=100, "Use Estimated Average Phasor"=FALSE} ("Phasor SDV Options"), Variant=w54) -> (data=w45:T2, error out=w44:errorcluster)
      n12 = call "Alligator Variables Storage.vi"("Get(F)/Set"=FALSE, "AlliGator Variable"=AlliGator_Variables_List."Source Image:ROIs" ("Alligator Variable"), "Error In"=w37) -> ("Error Out"=w106:errorcluster, "Data out"=w107:variant)  [unwired: 6 in, 1 out]
      n13 = Unbundle By Name(w40) -> ("Map Resolution X"=w39:i32, "Map Resolution Y"=w38:i32)
      n14 = case shown="0, Default" w56 {
        tunnel: [w112 w114] -> w65
        tunnel: w64 -> [w110 w114]
        tunnel: [w111 w113] -> w62
        tunnel: w63 -> [w109 w113]
        tunnel: w61 -> [w112 w116]
        tunnel: w60 -> [w111 w115]
        tunnel: [w112 w116] -> w50
        tunnel: [w111 w115] -> w49
        tunnel: [w110 w114] -> w48
        tunnel: [w109 w113] -> w47
        frame 0, Default {
        }
        frame 1 {
        }
      }
      n15 = Variant To Data(error in=w106, type=T6[] [] ("Stored ROIs in"), Variant=w107) -> (data=w69:T6[], error out=w101:errorcluster)
      n16 = call "AlliGator Get Pixel Count Constraints.vi"("error in (no error)"=w37) -> ("error out"=w102:errorcluster, "Pixel Count Constraints"=w103:T46)  [unwired: 9 in]
      n17 = Unbundle By Name(w45) -> ("Use Estimated Average Phasor"=w46:bool)
      n18 = call "AlliGator Is Full-Frame Single-Pixel Calibration.vi"("error in (no error)"=w37, "Map Resolution Y"=w38, "Map Resolution X"=w39) -> ("error out"=w36:errorcluster, "Full-Frame Single-Pixel Calibration?"=w35:bool)  [unwired: 7 in]
      n19 = call "AlliGator Get Sum Image Threshold.vi"("error in (no error)"=w102, "Pixel Counts Constraints"=w103, "Image in"=w65) -> ("error out"=w71:errorcluster, "Pixel Threshold Low"=w98:sgl, "Pixel Threshold High"=w99:sgl)  [unwired: 2 in, 4 out]
      n20 = Bundle By Name(cluster=cluster{"Image Sum":T5, "Image Array":T5[]} {"Image Sum"=refnum, "Image Array"=[]} ("Images"), "Image Sum"=w65, "Image Array"=w62) -> (w95:cluster{"Image Sum":T5, "Image Array":T5[]})
      n21 = Merge Errors(w36, w41, w71, w101, w97, w44, w43) -> (w100:errorcluster)
      n22 = call "AlliGator Phasor Frequency.vi"() -> ("Phasor Frequency"=w51:dbl[unit])
      n23 = Array Size(array=w69) -> (size(s)=w68:i32)
      n24 = Array Size(array=w62) -> (size(s)=w94:i32)
      n25 = case shown="1, Default" w68 {
        selector: w68 -> [_ w156]
        tunnel: w100 -> [_ w151]
        tunnel: w99 -> [_ w200]
        tunnel: w98 -> [_ w199]
        tunnel: w96 -> [_ w198]
        tunnel: w95 -> [_ w197]
        tunnel: w94 -> [_ w196]
        tunnel: w93 -> [_ w194]
        tunnel: [w117 w193] -> w92
        tunnel: w91 -> [w123 w192]
        tunnel: [w123 w191] -> w90
        tunnel: w89 -> [w122 w190]
        tunnel: [w122 w189] -> w88
        tunnel: w87 -> [w121 w188]
        tunnel: [w121 w187] -> w86
        tunnel: w85 -> [w120 w186]
        tunnel: w84 -> [w119 w184]
        tunnel: [w119 w183] -> w83
        tunnel: w82 -> [w124 w180]
        tunnel: [w124 w179] -> w81
        tunnel: w51 -> [_ w136]
        tunnel: [_ w176] -> w80
        tunnel: w79 -> [_ w175]
        tunnel: [w120 w174] -> w78
        tunnel: [_ w173] -> w77
        tunnel: [_ w170] -> w76
        tunnel: [_ w168] -> w75
        tunnel: w73 -> [_ w167]
        tunnel: w72 -> [_ w166]
        tunnel: w40 -> [_ w165]
        tunnel: w70 -> [_ w163]
        tunnel: w69 -> [_ w161]
        tunnel: [_ w154] -> w67
        tunnel: w59 -> [_ w140]
        tunnel: w45 -> [_ w137]
        tunnel: w46 -> [_ w135]
        tunnel: w42 -> [_ w131]
        tunnel: w35 -> [_ w130]
        frame 0 {
          n26 = One Button Dialog(message="All ROIs Phasor Analysis: no ROI defined!") -> ()  [unwired: 1 in, 1 out]
          n27 = xnode "Error Ring"() -> ("error out"=w117:errorcluster)
        }
        frame 1, Default {
          n28 = call "AlliGator Get Decay Time Axis v2.vi"("Number of Gates"=w196) -> ("t Array"=w195:dbl[unit][])  [unwired: 14 in]
          n29 = call "Embedded Progress Bar Q.vi"("Progress Bar Queue Name"="AlliGator Progress Bar Q") -> ("Progress Bar Queue"=w143:refnum<queue>)  [unwired: 6 in]
          n30 = call "AlliGator Get-Set Decay Preprocessing Parameters.vi"("Get (F)/Set"=FALSE, "Error In"=w151) -> ("Error Out"=w149:errorcluster, "Decay Preprocessing Parameters out"=w145:T39)  [unwired: 8 in]
          n31 = call "Logical Processors Used.vi"() -> ("# Logical Processor Used"=w132:i32)  [unwired: 6 in]
          n32 = call "Send Embedded Progress Bar Update.vi"("Max Iterations N"=w156, "Current Iteration i (i or -1: standard or || iteration; 0 or -2: first standard or || iteration)"=-2 ("Current Iteration i (-1: || iteration, -2: first || iteration)"), "Progress Bar Queue in"=w143) -> ("Error Out"=w159:errorcluster, "Progress Bar Queue out"=w160:refnum<queue>)  [unwired: 7 in]
          n33 = node(w195) -> (w164:dbl[])
          n34 = for {
            tunnel: w161 -> [w301] mode=indexing
            tunnel: w200 -> [w300]
            tunnel: w199 -> [w299]
            tunnel: w197 -> [w298]
            tunnel: w198 -> [w297]
            tunnel: [w272] -> w162
            tunnel: w164 -> [w284]
            tunnel: w194 -> [w285]
            tunnel: [w286] -> w182 mode=indexing if=w256
            tunnel: w136 -> [w296]
            tunnel: [w294] -> w152 mode=indexing if=w256
            tunnel: [w295] -> w172 mode=indexing if=w256
            tunnel: [w264] -> w185
            tunnel: [w293] -> w181 mode=indexing if=w256
            tunnel: [w292] -> w154 mode=indexing if=w256
            tunnel: [w283] -> w178
            tunnel: [w291] -> w177
            tunnel: [w290] -> w170 mode=indexing if=w279
            tunnel: w148 -> [w269]
            tunnel: [w282] -> w168
            tunnel: w167 -> [w289]
            tunnel: w166 -> [w288]
            tunnel: w165 -> [w287]
            tunnel: w163 -> [w281]
            tunnel: w156 -> [w280]
            tunnel: w159 -> [w276]
            tunnel: [w274] -> w157
            tunnel: w160 -> [w277]
            tunnel: [w275] -> w158
            tunnel: [FALSE ("Abort?")] -> w153
            tunnel: [w268] -> w150 mode=indexing
            tunnel: w145 -> [w271]
            tunnel: w140 -> [w267]
            tunnel: [w266] -> w139 mode=indexing if=w256
            tunnel: w137 -> [w262]
            tunnel: [w265] -> w138 mode=indexing if=w256
            tunnel: w135 -> [w263]
            tunnel: [w261] -> w134 mode=indexing
            tunnel: [w260] -> w133 mode=indexing
            workers-P: w132 -> [_]
            tunnel: w131 -> [w259]
            tunnel: w130 -> [w258]
            tunnel: [w257] -> w129 mode=indexing if=w256
            i -> [w264]
            n35 = global read "AlliGator Abort.vi" "Abort?"() -> (w272:bool)
            n36 = call "Send Embedded Progress Bar Update.vi"("Error In"=w276, "Current Iteration i (i or -1: standard or || iteration; 0 or -2: first standard or || iteration)"=-1 ("Current Iteration i (-1: || iteration, -2: first || iteration)"), "Progress Bar Queue in"=w277) -> ("Error Out"=w274:errorcluster, "Progress Bar Queue out"=w275:refnum<queue>)  [unwired: 7 in]
            n37 = case shown="False" w272 {
              tunnel: w301 -> [w356 _]
              tunnel: w300 -> [w355 _]
              tunnel: w299 -> [w354 _]
              tunnel: w298 -> [w353 _]
              tunnel: w297 -> [w352 _]
              tunnel: w269 -> [w351 _]
              tunnel: w296 -> [w318 _]
              tunnel: [w311 _] -> w295
              tunnel: [w312 _] -> w294
              tunnel: [w346 _] -> w293
              tunnel: [w345 _] -> w292
              tunnel: [w325 _] -> w291
              tunnel: [w344 _] -> w290
              tunnel: [w342 _] -> w256
              tunnel: w289 -> [w341 _]
              tunnel: w288 -> [w340 _]
              tunnel: w287 -> [w339 _]
              tunnel: [w338 _] -> w286
              tunnel: w285 -> [w335 _]
              tunnel: w284 -> [w334 _]
              tunnel: [w317 _] -> w283
              tunnel: [w329 _] -> w282
              tunnel: w281 -> [w313 _]
              tunnel: w280 -> [w328 _]
              tunnel: w264 -> [w306 _]
              tunnel: [w327 _] -> w278
              tunnel: [w324 _] -> w268
              tunnel: w271 -> [w326 _]
              tunnel: w267 -> [w322 _]
              tunnel: [w320 _] -> w266
              tunnel: [w310 _] -> w265
              tunnel: w263 -> [w309 _]
              tunnel: w262 -> [w308 _]
              tunnel: [w307 _] -> w261
              tunnel: [w305 _] -> w260
              tunnel: w259 -> [w304 _]
              tunnel: w258 -> [w303 _]
              tunnel: [w302 _] -> w257
              frame False {
                # "needed to allow pixel-to-pixel calibration\n(includes NaN + NaN i phasors)"
                n38 = Unbundle By Name(w356) -> ("ROI Descriptor"=w337:T7, "ROI Name"=w344:string)
                n39 = call "Keep String in Array.vi"("Current Index"=w306, "Number of Elements"=w328) -> ("Keep String"=w327:bool)  [unwired: 9 in]
                n40 = call "AlliGator Compute ROI Decay.vi"("Pixel Threshold High"=w355, "Loop ID"=w306, "Pixel Threshold Low"=w354, "error in (no error)"=w351, "Decay Peak  Constraints"=w352, "ROI Descriptor"=w337, "Images"=w353) -> ("error out"=w323:errorcluster, "# Valid Pixels"=w305:i32, "ROI Center"=w336:cluster{"X":i32, "Y":i32}, "Decay Points"=w333:dbl[])  [unwired: 1 out]
                n41 = Bundle(w334, "Decay Points"=w333) -> (w332:cluster{dbl[], "Decay Points":dbl[]})  [unwired: 1 in]
                n42 = call "AlliGator Preprocess Decay v3.vi"("Decay Preprocessing Parameters"=w326, "Error In"=w323, "Time-Gated Reference Decay"=w335, "# Pixels"=w305, "Decay (in)"=w332) -> ("Error Out"=w330:errorcluster, "Decay (out)"=w317:T49, "Decay Metadata"=w331:T10, "Message"=w329:string)  [unwired: 3 in]
                n43 = call "Phasor Compute Phasor from Decay v2.vi"("Error In"=w330, "Phasor Frequency"=w318, "Time-Gated Decay"=w317) -> ("Error Out"=w307:errorcluster, "s"=w349:dbl, "g"=w350:dbl, "Total Intensity"=w302:dbl)  [unwired: 4 in, 1 out]
                n44 = Bundle By Name(cluster=T1 {"g"=0.0, "s"=0.0} ("Phasor"), "g"=w350, "s"=w349) -> (w347:T1)
                n45 = Bundle By Name(cluster=w331, "ROI Center"=w336, "ROI Descriptor"=w337) -> (w338:T10)
                n46 = call "AlliGator Select Phasor Calibration v3.vi"("Calibration Phasor"=w341, "ROI Center (Default: undefined)"=w336, "Basic Calibration Options"=w304, "Calibration Phasor Series"=w340, "Phasor Calibration Map"=w339, "Calibration Map MD5 Digest"=w322, "Error In"=w307, "Current Data Set (-1: single)"=w313, "Full-Frame Single-Pixel Calibration?"=w303) -> ("Calibration Phasor"=w320:T16, "Error Out"=w319:errorcluster)  [unwired: 4 in, 1 out]
                n47 = call "Tiny Clear Error.vi"("Error In"=w319) -> ("no Error Out"=w314:errorcluster)  [unwired: 8 in]
                n48 = Unbundle By Name(w314) -> ("status"=w343:bool)
                n49 = call "Phasor Compute Standard Deviation (Poisson).vi"("Time-Gated Decay"=w317, "Phasor SDV Options in"=w308, "Phasor Frequency"=w318, "Error In"=w314, "Calibration Phasor (m, phi)"=w320) -> ("(Mean) Phasor (g, s)"=w311:T1, "Phasor SDV (g, s)"=w310:T1, "Calibrated (Mean) Phasor (g, s)"=w316:T1)  [unwired: 4 in, 4 out]
                n50 = call "Phasor Calibration v3.vi"("Compute Lifetimes? (F)"=TRUE ("Init?"), "Error In"=w314, "Phasor Frequency"=w318, "Calibration Phasor"=w320, "Measured Phasor"=w347) -> ("Error Out"=w324:errorcluster, "Calibrated Phase Lifetime"=w325:dbl[unit], "Calibrated Phasor"=w315:T1)  [unwired: 1 in, 3 out]
                n51 = Not(x=w343) -> (.not. x?=w342:bool)
                n52 = Select(t=w316, s=w309, f=w315) -> (s? t:f=w312:T1)
                n53 = Unbundle By Name(w312) -> ("g"=w346:dbl, "s"=w345:dbl)
              }
              frame True {
              }
            }
            n54 = Compound Arithmetic op=AND(w256, w278) -> (w279:bool)
          }
          n55 = flat-sequence {
            tunnel: w136 -> [w205]
            tunnel: w149 -> [w203]
            tunnel: [w202] -> w148
            frame #0 {
              (unwired) TRUE ("want seconds? (F)")
              n56 = node(w205) -> (w204:dbl)
              n57 = call "Get Notebook Queue.vi"() -> ("Notebook Queue"=w206:refnum<queue>)  [unwired: 9 in]
              n58 = call "Current Date & Time String (High Precision).vi"() -> ("time string"=w210:string, "date string"=w209:string)  [unwired: 8 in, 2 out]
              n59 = Format Into String(format string="All ROIs Phasor Analysis (non-interactive) Started on %s at %s\nf = %#g MHz", error in=w203, w209, w210, w204) -> (resulting string=w211:string, error out=w212:errorcluster)  [unwired: 1 in]
              n60 = call "Get Current Message Text Format.vi"("Text Format"=Text_Format_List."Result") -> ("Message Formatting"=w208:T50)  [unwired: 8 in, 1 out]
              n61 = call "Send Message to Notebook.vi"("Text Formatting"=w208, "Error In"=w212, "Text"=w211, "Notebook Queue"=w206) -> ("Error Out"=w202:errorcluster)  [unwired: 4 in, 1 out]
            }
          }
          n62 = global write "AlliGator Abort.vi" "Abort?"(w153) -> ()
          n63 = Empty Array?(array=w152) -> (empty?=w169:bool)
          n64 = call "Send Embedded Progress Bar Update.vi"("Stop Progress Bar (F)"=TRUE ("Hide Progress Bar (F)"), "Error In"=w157, "Progress Bar Queue in"=w158) -> ("Error Out"=w155:errorcluster)  [unwired: 7 in, 1 out]
          n65 = Compound Arithmetic op=OR(w169, w162) -> (w171:bool)
          n66 = Merge Errors(w150) -> (w147:errorcluster)
          n67 = case shown="False" w171 {
            tunnel: [w217 w238] -> w193
            tunnel: w192 -> [_ w247]
            tunnel: [w236 w247] -> w191
            tunnel: w190 -> [_ w241]
            tunnel: [w219 w241] -> w189
            tunnel: w188 -> [w230 w246]
            tunnel: [w229 w246] -> w187
            tunnel: w186 -> [_ w245]
            tunnel: [w232 w245] -> w174
            tunnel: w152 -> [w235 _]
            tunnel: w172 -> [w222 _]
            tunnel: w185 -> [w223 _]
            tunnel: w184 -> [_ w244]
            tunnel: [w224 w244] -> w183
            tunnel: w182 -> [w225 _]
            tunnel: w181 -> [w234 _]
            tunnel: w154 -> [w233 _]
            tunnel: w180 -> [_ w243]
            tunnel: [w231 w243] -> w179
            tunnel: w178 -> [w231 _]
            tunnel: w136 -> [w227 _]
            tunnel: w177 -> [w221 _]
            tunnel: [w221 dbl[unit] nan ("Calibrated Lifetime")] -> w176
            tunnel: w175 -> [w220 _]
            tunnel: [w219 w241] -> w173
            tunnel: w162 -> [_ w240]
            tunnel: w155 -> [_ _]
            tunnel: w147 -> [w218 _]
            tunnel: w139 -> [w216 _]
            tunnel: w137 -> [w215 _]
            tunnel: w138 -> [w214 _]
            tunnel: w134 -> [_ _]
            tunnel: w133 -> [_ _]
            tunnel: w129 -> [w213 _]
            frame False {
              n68 = call "Tiny Clear Error.vi"("Error In"=w218) -> ("no Error Out"=w217:errorcluster)  [unwired: 8 in]
              n69 = Bundle By Name(cluster=T9 {"Phasor Plot Name"="", "Raw Phasor Plot"=[], "Phasor Frequency"=160000000.0, "[Decay Metadata]"=[], "Raw Phasor Plot SDV"=[], "Phasor SDV Options"={"Compute Estimated SDV"=FALSE, "# Replicas"=100, "Use Estimated Average Phasor"=FALSE}, "[Calibration Phasor]"=[], "Intensity Array"=[]} ("array"), "Phasor Frequency"=w227, "Raw Phasor Plot"=w222, "[Decay Metadata]"=w225, "Phasor Plot Name"=w220, "Raw Phasor Plot SDV"=w214, "Phasor SDV Options"=w215, "[Calibration Phasor]"=w216, "Intensity Array"=w213) -> (w226:T9)
              n70 = Bundle(w234, w233) -> (w232:cluster{dbl[], dbl[]})  [unwired: 1 in]
              n71 = Index Array(array=w235, index=w223) -> (element=w219:T1)
              n72 = Index Array(array=w222, index=w223) -> (element=w236:T1)
              n73 = Index Array(array=w225, index=w223) -> (element=w224:T10)
              n74 = Build Array (concatenate)(w230, w226) -> (w229:T9[])
            }
            frame True {
              n75 = xnode "Error Ring"() -> ("error out"=w239:errorcluster)
              n76 = xnode "Error Ring"() -> ("error out"=w237:errorcluster)
              n77 = Select(t=w239, s=w240, f=w237) -> (s? t:f=w238:errorcluster)
            }
          }
        }
      }
      n78 = in-place-cluster #2("Current Dataset Images 1.SGL Sum Image"=w50, "Current Dataset Images 1.SGL Gate Images"=w49, "Current Dataset Images 2.SGL Sum Image"=w48, "Current Dataset Images 2.SGL Gate Images"=w47, "Reference Decay"=w93, "ROI Decay"=w81, "Calibration Phasor"=w73, "Calibration Phasor Series"=w72, "Last Raw Phasor"=w90, "Last Calibrated Phasor"=w88, "[Phasor Graph:Raw Phasor Plots]"=w86, "Phasor Graph:Phasor Plot"=w78, "Decay  Metadata"=w83, "Phasor Calibration Map"=w40, "Current Dataset"=w70, "Calibration Map MD5 Digest"=w59) -> (w33:T17)
      n79 = call "Add Line Feed to String.vi"("String"=w75) -> ("String\\n"=w74:string)  [unwired: 8 in]
    }
    n80 = in-place-dvr #1(w33) -> (→"AlliGator Internal Variables DVR":refnum<data-value>)  [unwired: 1 out]
  }
  "Calibrated Phase Lifetime" <- w20
  "Phasor Plot" <- w18
  "Calibrated Phasor" <- w17
  n81 = call "High Resolution Timing.vi"("relative seconds (NaN)"=w13, "Error In"=w4) -> ("elapsed (relative) seconds"=w12:dbl, "Error Out"=w5:errorcluster)  [unwired: 15 in, 1 out]
  n82 = Array Size(array=w3) -> (size(s)=w8:i32)
  n83 = call "Concatenate String Array.vi"("Max Number of Elements (None: -1)"=8 ("Max Number of Elements (None: 1)"), "Separator (TAB)"=", ", "String Array"=w9) -> ("Formatted String"=w10:string)  [unwired: 8 in]
  n84 = call "Current Date & Time String (High Precision).vi"("Error In"=w5) -> ("Error Out"=w2:errorcluster, "on <Date> at <Time>"=w1:string)  [unwired: 7 in, 2 out]
  n85 = case shown="1, Default" w8 {
    selector: w8 -> [_ w361]
    tunnel: w1 -> [_ w367]
    tunnel: [w357 w366] -> w14
    tunnel: w12 -> [_ w364]
    tunnel: ["No valid ROIs to process..." w363] -> w11
    tunnel: w10 -> [_ w362]
    tunnel: w6 -> [_ w360]
    tunnel: w2 -> [w357 w359]
    frame 0 {
    }
    frame 1, Default {
      n86 = Format Into String(format string="All ROIs Phasor Analysis (%d):\n%s\n%scompleted %s\nCPU: %#g s", error in=w359, w361, w362, w360, w367, w364) -> (resulting string=w363:string, error out=w366:errorcluster)  [unwired: 1 in]
    }
  }
  "error out" <- w14
  "Message" <- w11
